vi "Sub Super Duper_2014 05 30_JWb.vi"(0 "VISA resource name":refnum<visa-resource-name>="GPIB0::17::INSTR", 1 "Sample Properties:":T9 {"Date Created" format="%<%Y/%m/%d>T"}, 2 "Gated SMU4 is...":bool, 3 "TRF Cluster":T10={"Step 4"=-38.0, "# of Loops"=1.0, "Transfer 2"=FALSE, "Start 4"=-2.0, "Total Points 2"=2, "Start 3"=40.0, "Stop 2"=-40.0, "Step 3"=-1.0, "Loop Step"=0.0, "Integration Time 3"=0, "Loop Wait"=0.0, "First Step"=0.0} {"Loop Wait" format="%<%H:%M:%S>t"; "Integration Time 3" scale=0.0..2.0; "Step 3" format="%.2f"; "Stop 2" format="%.2f"; "Start 3" format="%.2f"; "Start 4" format="%.2f"; "Step 4" format="%.2f"}, 4 "TSP Cluster":T11={"Transport"=FALSE, "Start 2"=0.0, "Stop 3"=-60.0, "Step 2"=-1.0, "Start"=0.0, "Step"=-10.0, "Total Points"=7, "Integration Time"=0} {"Integration Time" scale=0.0..2.0; "Step" format="%.2f"; "Start" format="%.2f"; "Step 2" format="%.2f"; "Stop 3" format="%.2f"; "Start 2" format="%.2f"}, 5 "Compliance Cluster":T6={"Var1 sweep settings"={"sweep spacing (linear: 0)"=0, "sweep mode"=FALSE, "compliance (V)"=100.0, "compliance (A)"=0.001}, "Var1 sweep settings 2"={"sweep spacing (linear: 0)"=0, "sweep mode"=FALSE, "compliance (V)"=100.0, "compliance (A)"=0.001}, "Var2 step settings 2"={"compliance (A)"=0.001, "compliance (V)"=100.0}, "Var2 step settings"={"compliance (A)"=0.001, "compliance (V)"=100.0}} {"Var2 step settings"."compliance (V)" format="%.2f"; "Var2 step settings"."compliance (A)" format="%^.2e"; "Var2 step settings 2"."compliance (V)" format="%.2f"; "Var2 step settings 2"."compliance (A)" format="%^.2e"; "Var1 sweep settings 2"."compliance (A)" format="%^.2e"; "Var1 sweep settings 2"."compliance (V)" format="%.2f"; "Var1 sweep settings 2"."sweep spacing (linear: 0)" items=["linear", "log 10", "log 25", "log 50"]; "Var1 sweep settings"."compliance (A)" format="%^.2e"; "Var1 sweep settings"."compliance (V)" format="%.2f"; "Var1 sweep settings"."sweep spacing (linear: 0)" items=["linear", "log 10", "log 25", "log 50"]}, 6 "Light Bathe Cluster":T2={"TG to BG:  "=FALSE, "TG to BG Durration"=120.0, "TRF to TSP:   "=FALSE, "TRF to TSP Duration"=120.0, "Post Measure: "=FALSE, "TG to BG (TSP):"=FALSE, "TG to BG Durration 3"=120.0} {"TG to BG Durration 3" format="%<%H:%M:%S>t"; "TRF to TSP Duration" format="%<%H:%M:%S>t"; "TG to BG Durration" format="%<%H:%M:%S>t"}, 7 "error in":errorcluster, 8 "Saved Folder:":path=path "C:/1DATA/2011", 9 "Wait Cluster":T5 {"Wait Time (s)" format="%.1g"; "Wait Countdown" format="%<%H:%M:%S%1u>t"}, 11 "TG Dielectric Prop":T1, 13 "Stop \nCountdown":bool, 15 "Loop Count":dbl, 16 "Gate Current Cluster":T3={"Gate Current (TSP)"={"Y2 axis on/off"=FALSE, "MINIMUM"=0.0, "MAXIMUM"=1.0, "Variable name"="Ig", "LIN or LOG axis"="LIN"}, "Gate Current (TRF)"={"Y2 axis on/off"=FALSE, "MINIMUM"=0.0, "MAXIMUM"=1.0, "Variable name"="Ig", "LIN or LOG axis"="LIN"}} {"Gate Current (TSP)"."MAXIMUM" format="%.9f"; "Gate Current (TSP)"."MINIMUM" format="%.9f"; "Gate Current (TRF)"."MAXIMUM" format="%.9f"; "Gate Current (TRF)"."MINIMUM" format="%.9f"}, 17 "Dielectric Constant (BG)":dbl) -> (12 "Status Indicator":bool, 14 "Vt Cluster":T4 {"Id Max" format="%.3g"; "Vt Max" format="%.3g"; "Vt Min" format="%.3g"; "Vt Ratio" format="%.3g"}, 20 "VISA resource name out":refnum<visa-resource-name>, 21 "TRF Path":path, 23 "TSP Path":path, 24 "Graph Cluster":T7, 25 "Char Cluster":T8 {"Mobility-Lin" format="%#_4e"; "On/Off" format="%#_4e"; "Mobility-Sat" format="%#_4e"}, 27 "error out":errorcluster)   [LabVIEW 2012]
uses:
  <vilib>/Platform/TimedLoop/XDataNode/wakeup.ctl
  <vilib>/Platform/TimedLoop/XDataNode/XDNodeRunTimeDep.lvlib
  <vilib>/Platform/TimedLoop/XDataNode/nitl_modes.ctl
  <vilib>/Platform/TimedLoop/XDataNode/timing_clust.ctl
  <vilib>/Platform/TimedLoop/XDataNode/XDataNode.xnode
panel:
  in  "Ambient Temp (Y/N) 2":bool=TRUE
  in  "Ambient Temp (Y/N)":bool=TRUE
  out "LKG Path":path
  # "Vg Sweep"
  # "Vd Step"
  # "Loops and Integration Time"
  # "Device Characteristics"
  # "Light Bath is..."
  # "Duration (hh:mm:ss)"
  # "Sample Properties:"
  # "%"
  # "nm"
  # "Device Properties:"
  # "um"
  # "um"
  # "Vg Step"
  # "Vd Step"
  # "Integration Time"
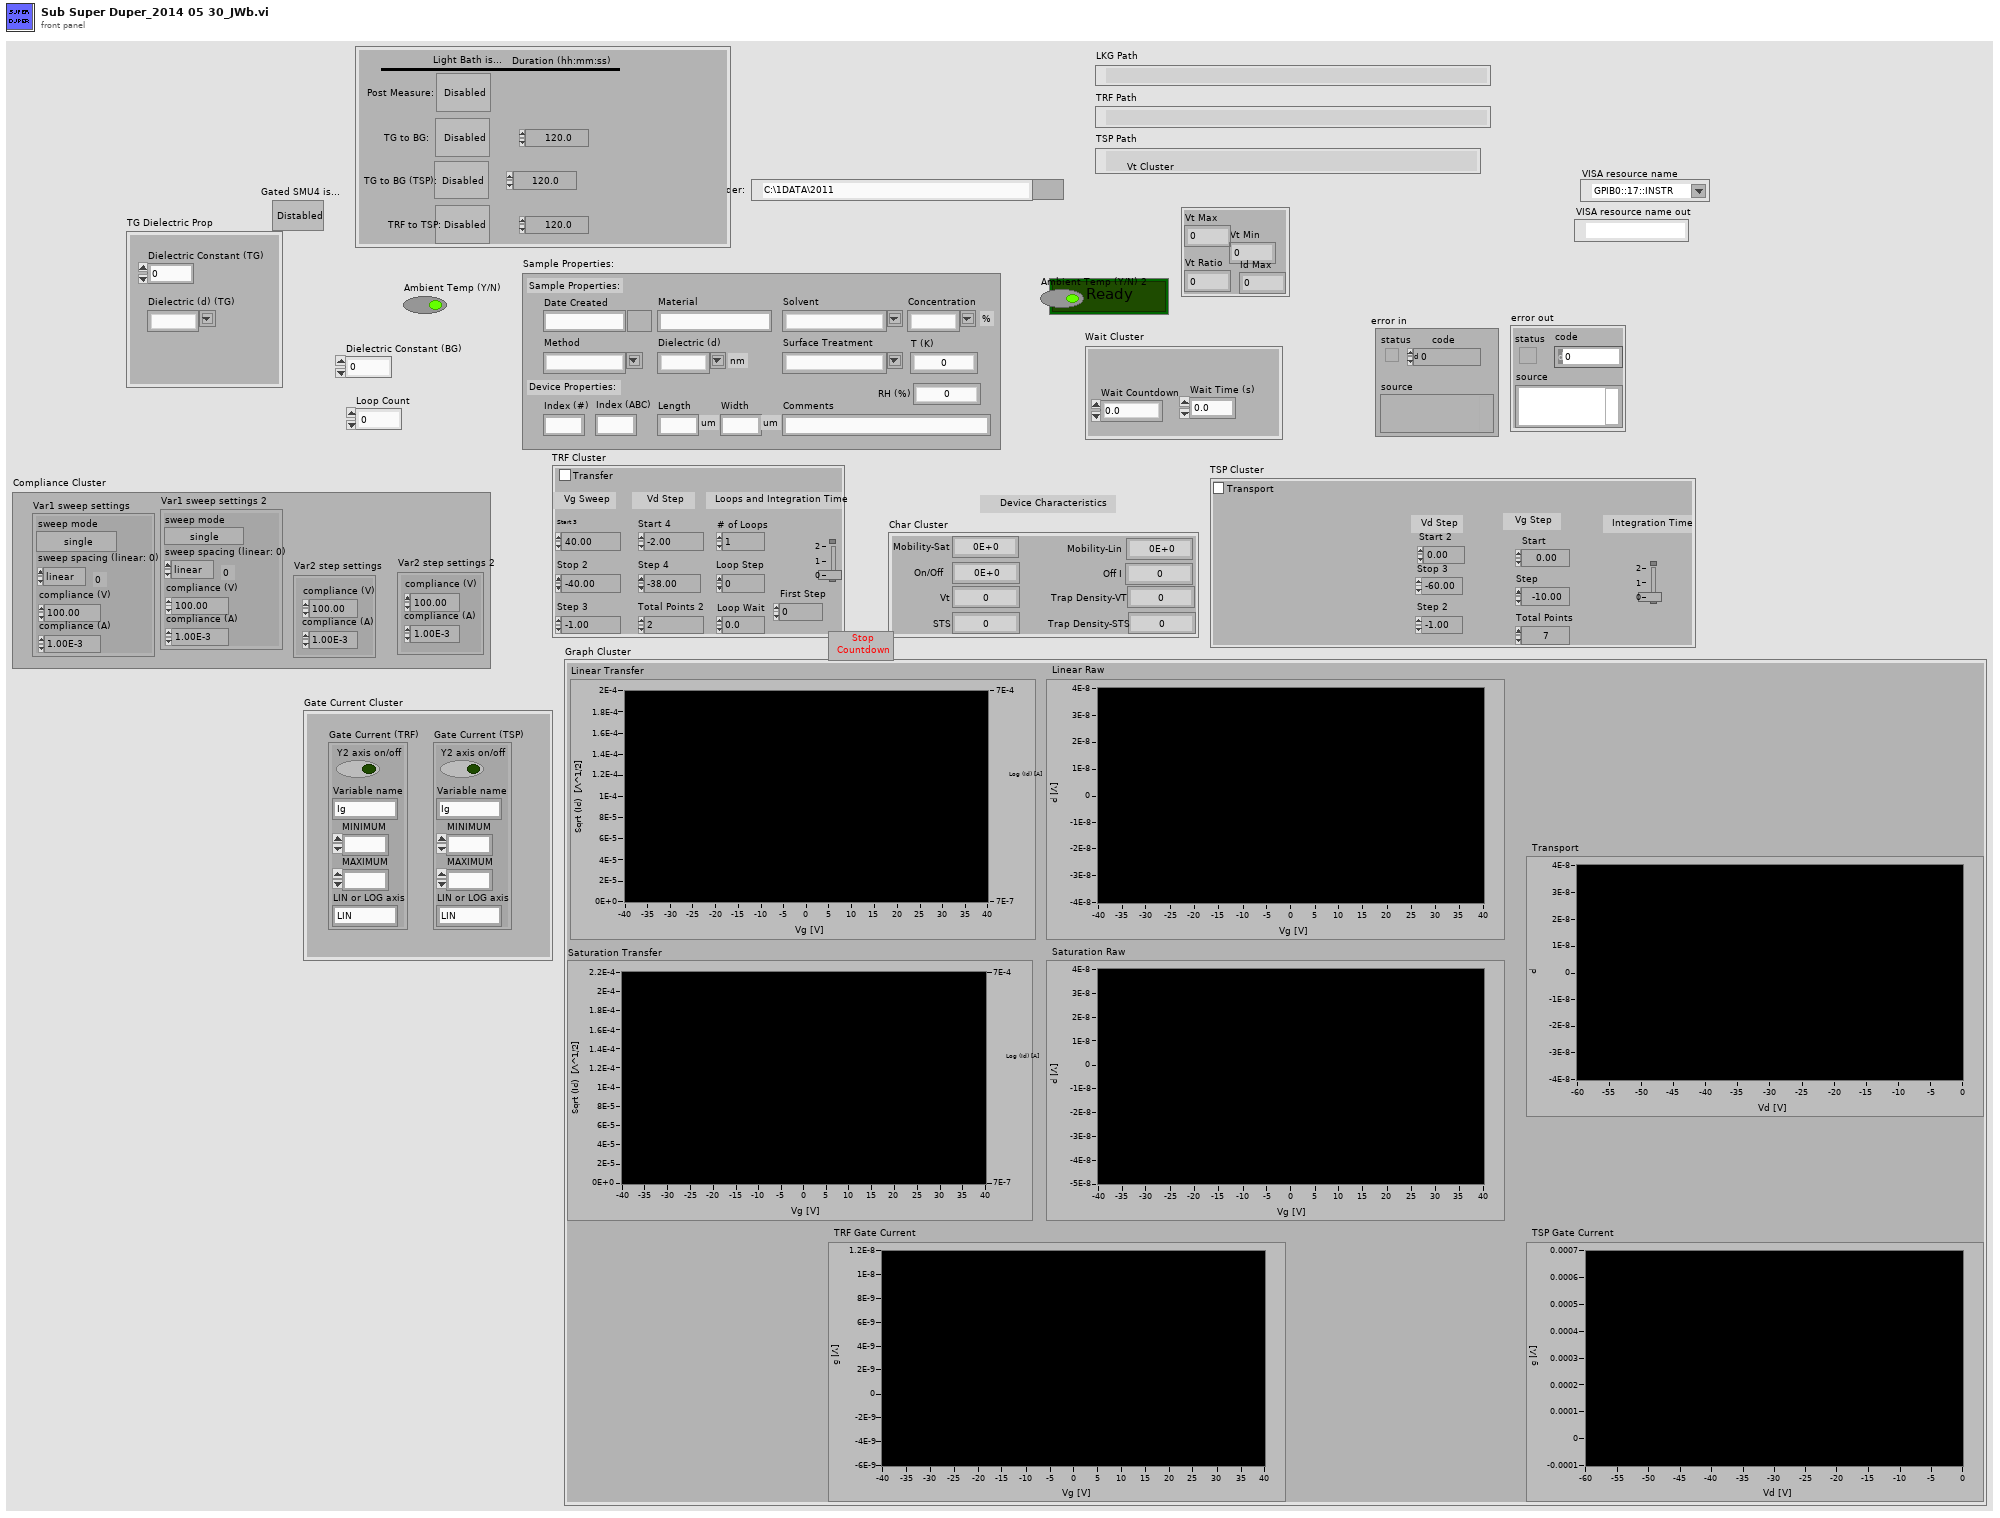
[diagram p1: front panel]
types:
  T1 = cluster{"Dielectric Constant (TG)":dbl, "Dielectric (d) (TG)":string}
  T2 = cluster{"TG to BG:  ":bool, "TG to BG Durration":dbl, "TRF to TSP:   ":bool, "TRF to TSP Duration":dbl, "Post Measure: ":bool, "TG to BG (TSP):":bool, "TG to BG Durration 3":dbl}
  T3 = cluster{"Gate Current (TSP)":cluster{"Y2 axis on/off":bool, "MINIMUM":ext, "MAXIMUM":ext, "Variable name":string, "LIN or LOG axis":string}, "Gate Current (TRF)":cluster{"Y2 axis on/off":bool, "MINIMUM":ext, "MAXIMUM":ext, "Variable name":string, "LIN or LOG axis":string}}
  T4 = cluster{"Vt Max":i32, "Vt Min":i32, "Vt Ratio":i32, "Id Max":i32}
  T5 = cluster{"Wait Countdown":dbl, "Wait Time (s)":dbl}
  T6 = cluster{"Var1 sweep settings":cluster{"sweep spacing (linear: 0)":u16, "sweep mode":bool, "compliance (V)":dbl, "compliance (A)":dbl}, "Var1 sweep settings 2":cluster{"sweep spacing (linear: 0)":u16, "sweep mode":bool, "compliance (V)":dbl, "compliance (A)":dbl}, "Var2 step settings 2":cluster{"compliance (A)":dbl, "compliance (V)":dbl}, "Var2 step settings":cluster{"compliance (A)":dbl, "compliance (V)":dbl}}
  T7 = cluster{"Linear Transfer":cluster{dbl[], "trace":dbl[]}[], "Linear Raw":cluster{dbl[], dbl[]}[], "Saturation Transfer":cluster{dbl[], "trace":dbl[]}[], "Saturation Raw":cluster{dbl[], dbl[]}[], "Transport":cluster{dbl[], dbl[]}[], "TRF Gate Current":cluster{dbl[], dbl[]}[], "TSP Gate Current":cluster{dbl[], dbl[]}[]}
  T8 = cluster{"Mobility-Sat":dbl, "Mobility-Lin":dbl, "On/Off ":dbl, "Off I":dbl, "Vt":dbl, "STS":dbl, "Trap Density-VT":dbl, "Trap Density-STS":dbl}
  T9 = cluster{"Date Created":timestamp, "Material":string, "Solvent":string, "Concentration":string, "Method":string, "Dielectric (d)":string, "Index (#)":string, "Index (ABC)":string, "Length":string, "Width":string, "Surface Treatment":string, "Comments":string, "T (K)":dbl, "RH (%)":dbl}
  T10 = cluster{"Step 4":dbl, "# of Loops":dbl, "Transfer 2":bool, "Start 4":dbl, "Total Points 2":u16, "Start 3":dbl, "Stop 2":dbl, "Step 3":dbl, "Loop Step":dbl, "Integration Time 3":u32, "Loop Wait":dbl, "First Step":dbl}
  T11 = cluster{"Transport":bool, "Start 2":dbl, "Stop 3":dbl, "Step 2":dbl, "Start":dbl, "Step":dbl, "Total Points":u16, "Integration Time":u32}
  T12 = cluster{"Vname":string, "Vname 2":string, "Vname 3":string, "Vname 4":string, "Iname":string, "Iname 2":string, "Iname 3":string, "Iname 4":string, "Mode":u16, "Mode 2":u16, "Mode 3":u16, "Mode 4":u16, "Function":u16, "Function 2":u16, "Function 3":u16, "Function 4":u16, "Value (V or A)":dbl, "Value (Either V or A) 2":dbl, "Value (Either V or A) 3":dbl, "Value (Either V or A) 4":dbl}
  T13 = typedef "XDNodeRunTimeDep.lvlib/timing_clust.ctl" = cluster{"Expected End [f-1]":u64, "Actual End [f-1]":u64, "Finished Late? [f-1]":bool, "Expected End [i-1]":u64, "Actual End [i-1]":u64, "Finished Late? [i-1]":bool, "Expected Start [i]":u64, "Actual Start [i]":u64, "Expected Start [f]":u64, "Actual Start [f]":u64, "Source Name":string, "Structure Name":string, "Period":i64, "Deadline":i64, "Offset":i64, "Start":i64, "Priority":i32, "Timeout":i32, "Mode":T14, "Wakeup Reason":T15, "Error":errorcluster, "Source Type":string, "Secondary Source Type":string, "Global End Time":u64, "Global Start Time":u64, "Frame Duration":u64, "Iteration Duration":u64, "Assigned CPU":i32, "I/O Scan Engine Mode":u32}
  T14 = typedef "XDNodeRunTimeDep.lvlib/nitl_modes.ctl" = enum32{"No Change", "Process missed periods, maintain original phase", "Discard missed periods, maintain original phase", "Process missed periods, ignore original phase", "Discard missed periods, ignore original phase"}
  T15 = typedef "XDNodeRunTimeDep.lvlib/wakeup.ctl" = enum32{"Normal", "Aborted", "Asynchronous wakeup", "Timing source error", "Timed loop error", "Timeout"}
  T16 = cluster{"Vt Max":i32, "Vt Min":i32, "Vt Ratio":i32, "Id Max":dbl}
  T17 = cluster{"Mobility-Sat":dbl, "Mobility-Lin":dbl, "On/Off Current":dbl, "Off I":dbl, "Vt":dbl, "STS":dbl, "Trap Density-VT":dbl, "Trap Density-STS":dbl}
  T18 = cluster{"sweep spacing (linear: 0)":u16, "sweep mode":bool, "compliance (V)":dbl, "compliance (A)":dbl}
  T19 = cluster{"compliance (A)":dbl, "compliance (V)":dbl}
  T20 = cluster{"Y2 axis on/off":bool, "MINIMUM":ext, "MAXIMUM":ext, "Variable name":string, "LIN or LOG axis":string}
  T21 = cluster{"Start 2":dbl, "Stop 3":dbl, "Step 2":dbl, "sweep spacing (linear: 0)":u16, "sweep mode":bool, "compliance (V)":dbl, "compliance (A)":dbl}
  T22 = cluster{"compliance (A)":dbl, "compliance (V)":dbl, "Start":dbl, "Total Points":u16, "Step":dbl}
  T23 = cluster{"Transport":cluster{dbl[], dbl[]}[], "Gate Current":cluster{dbl[], dbl[]}[]}
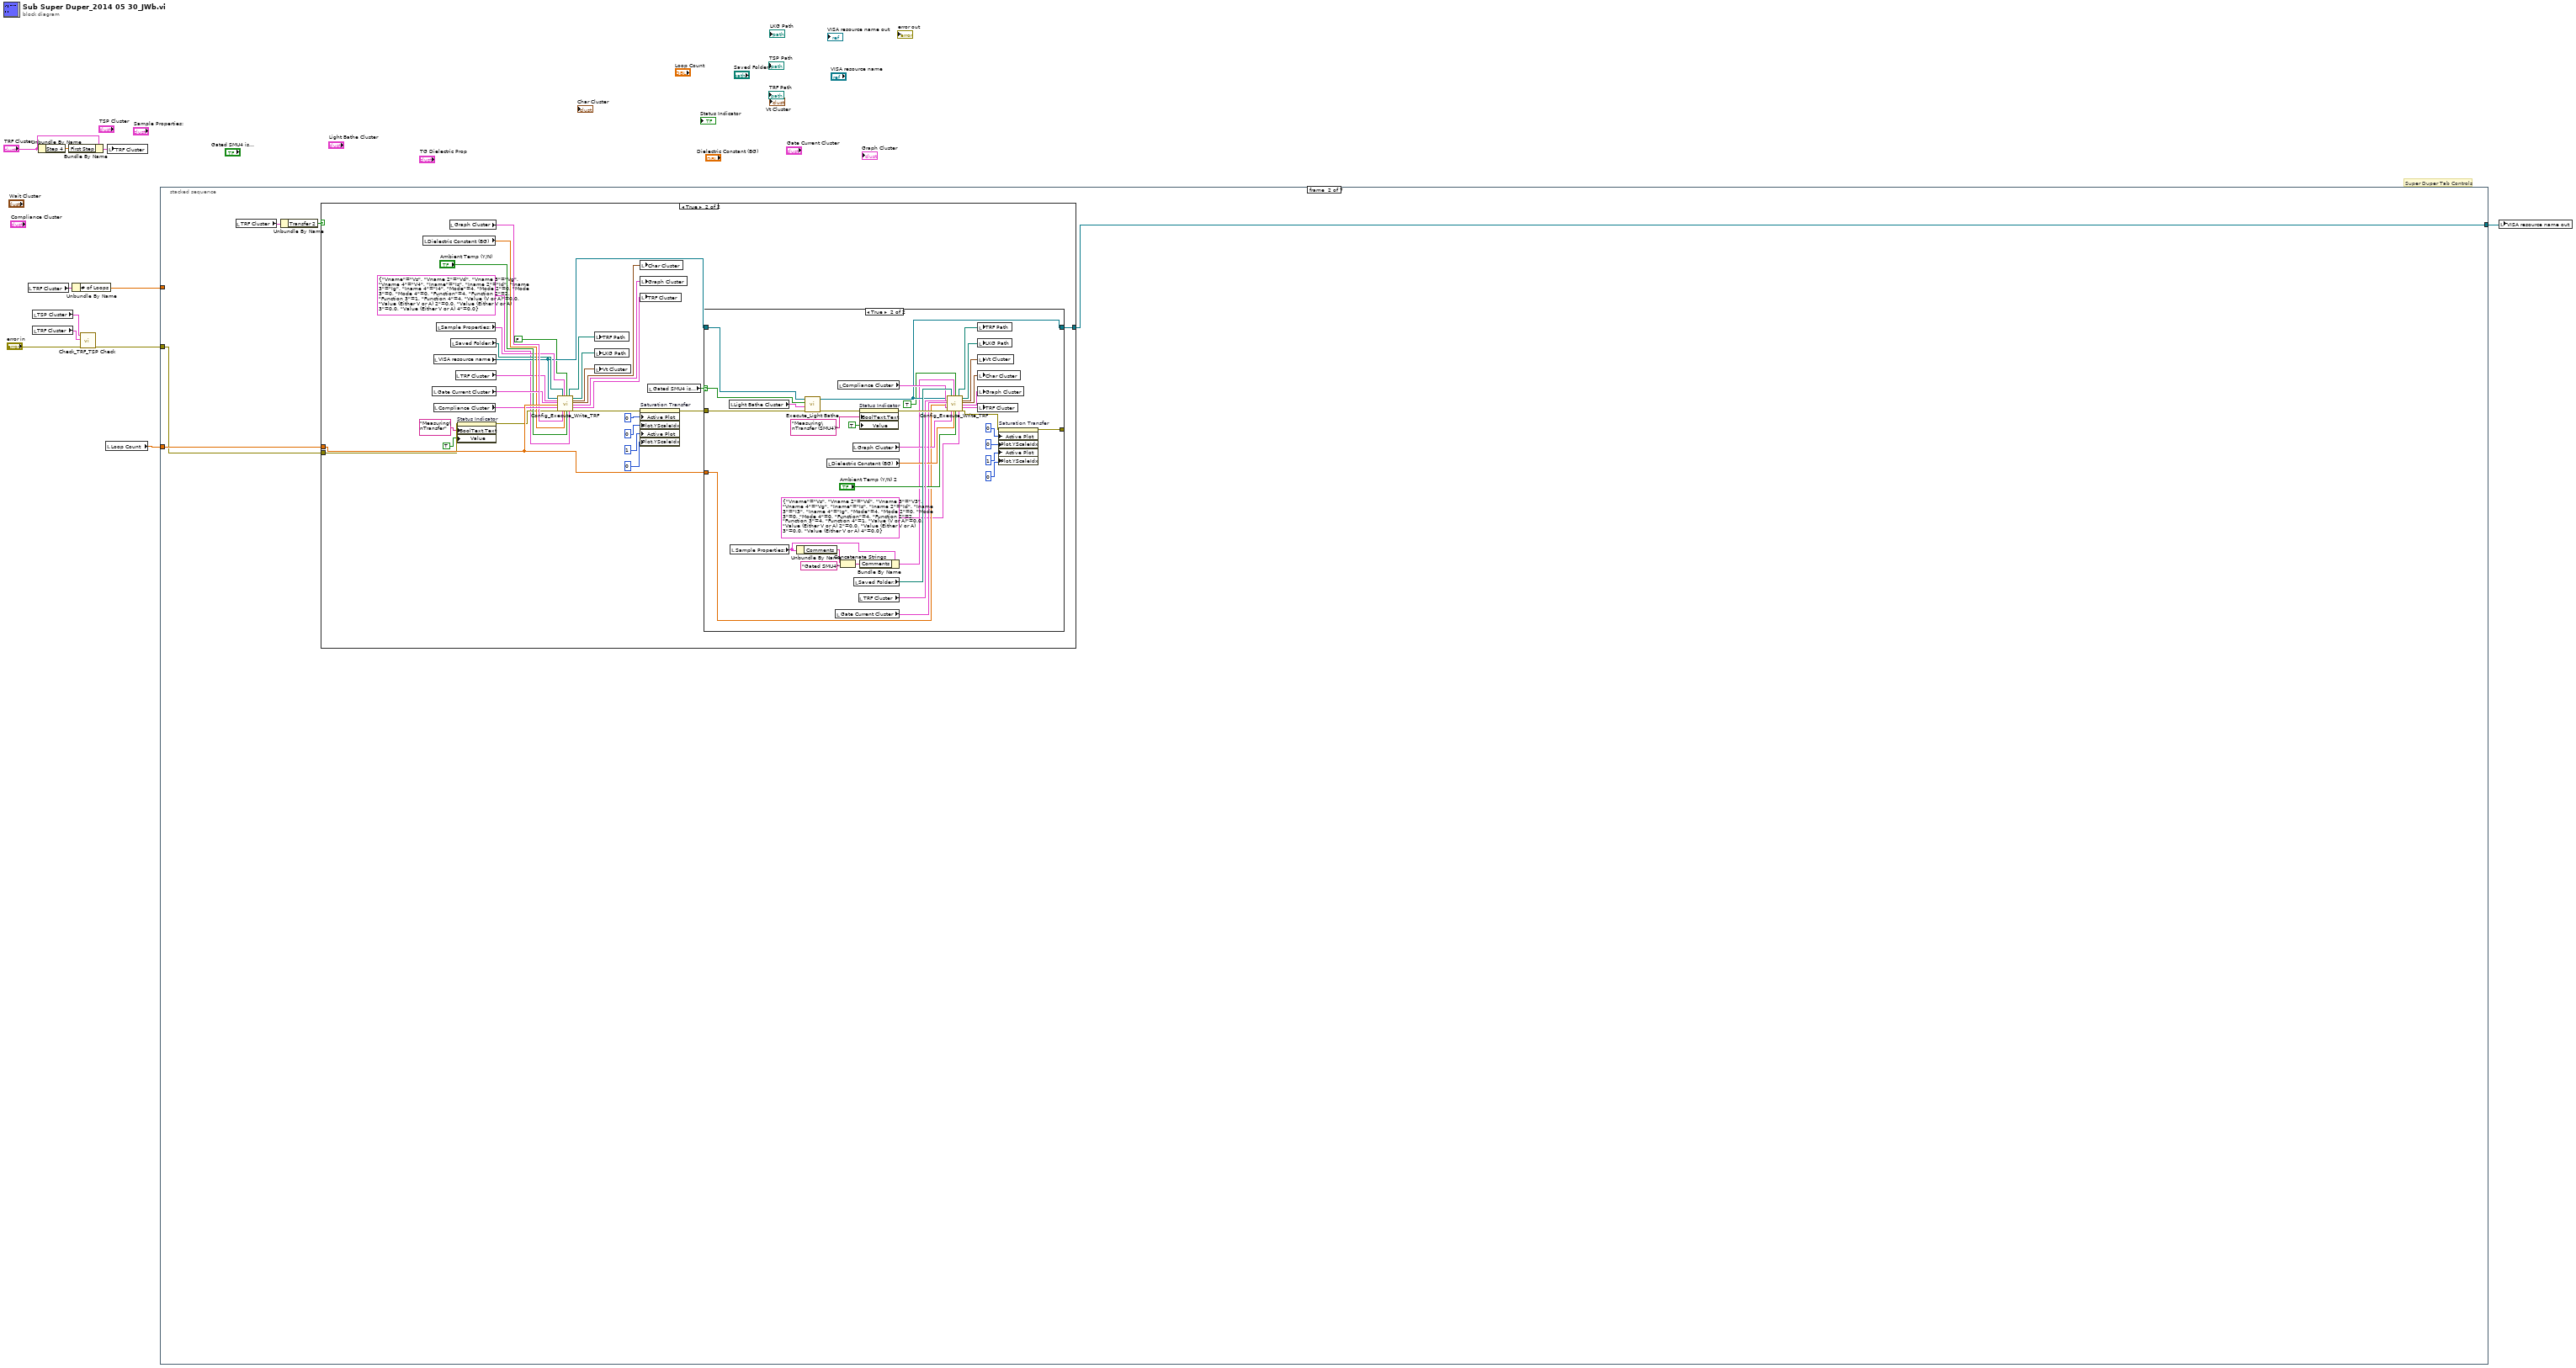
[diagram p0: block diagram]
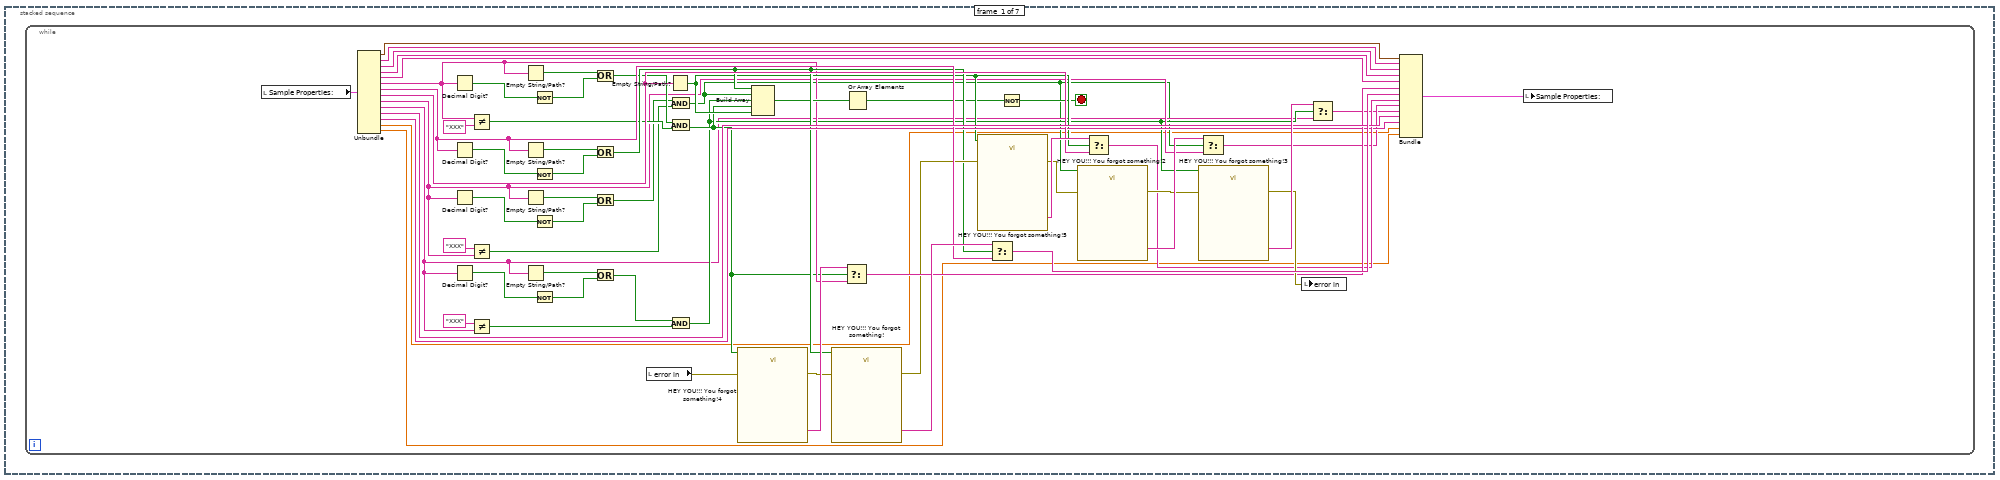
[diagram p2: hidden frame]
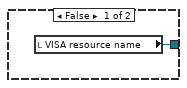
[diagram p3: hidden frame]
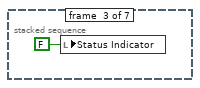
[diagram p5: hidden frame]
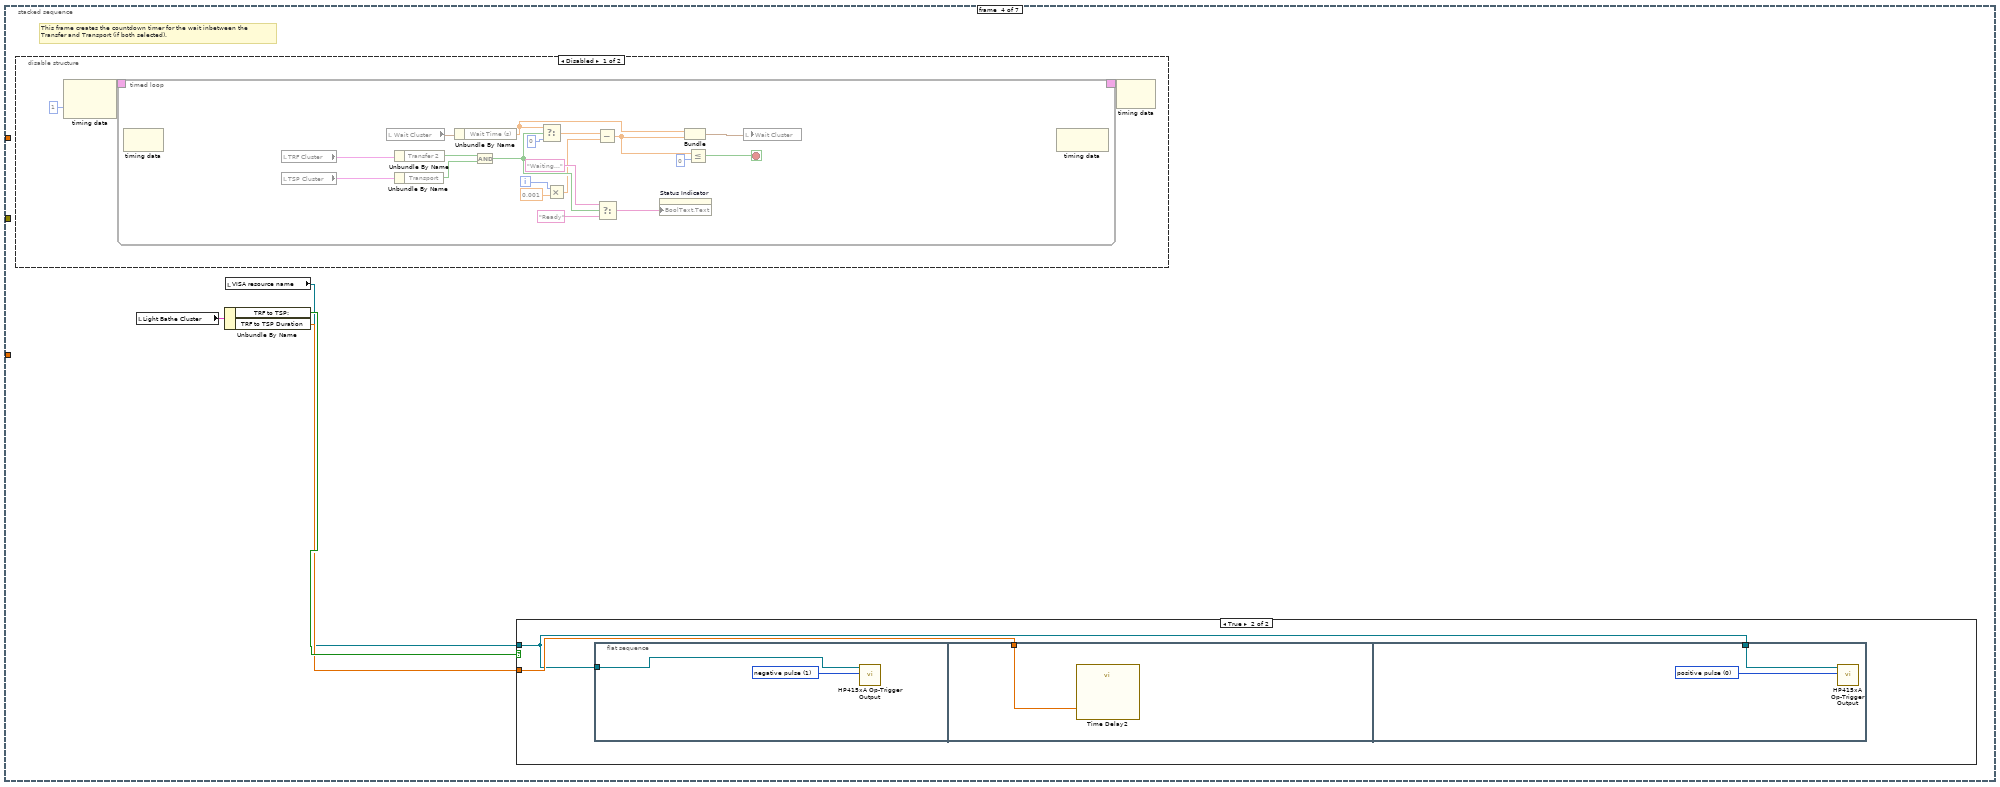
[diagram p6: hidden frame]
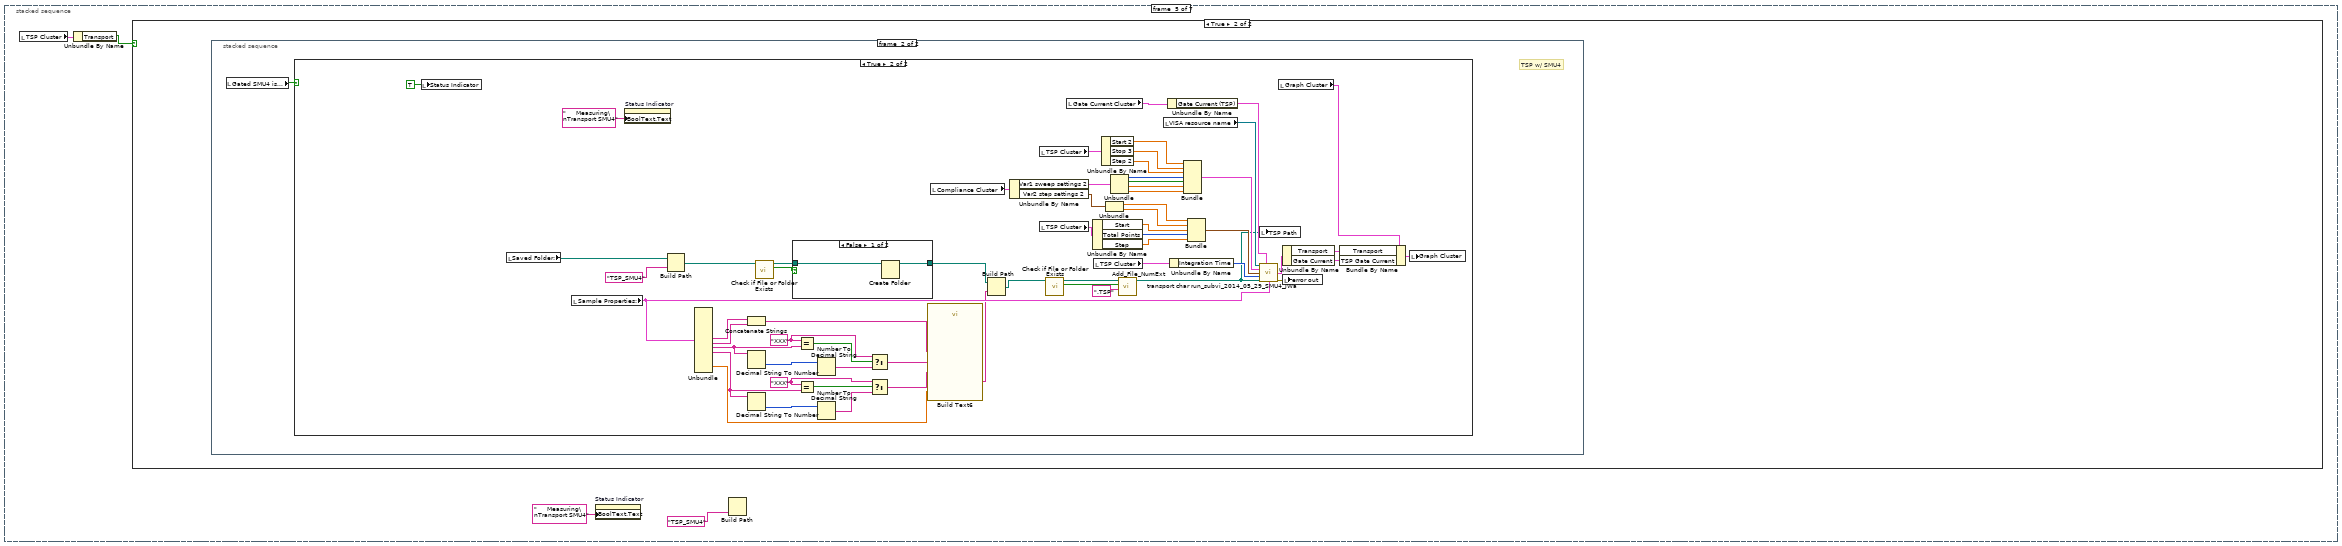
[diagram p9: hidden frame]
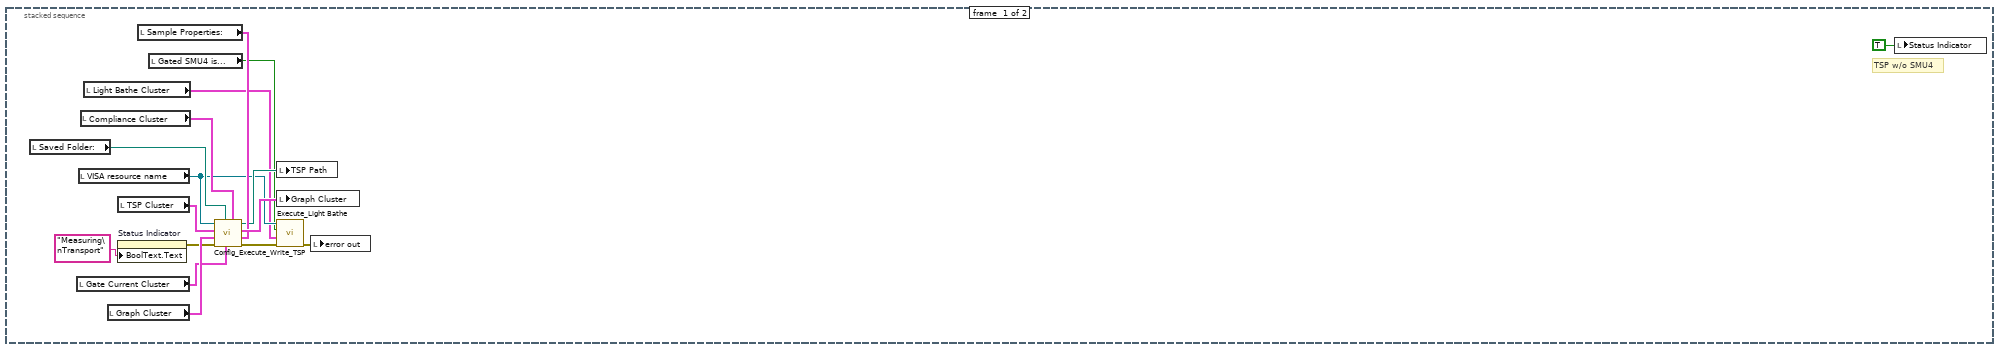
[diagram p11: hidden frame]
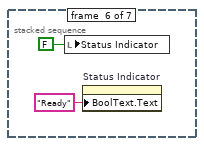
[diagram p14: hidden frame]
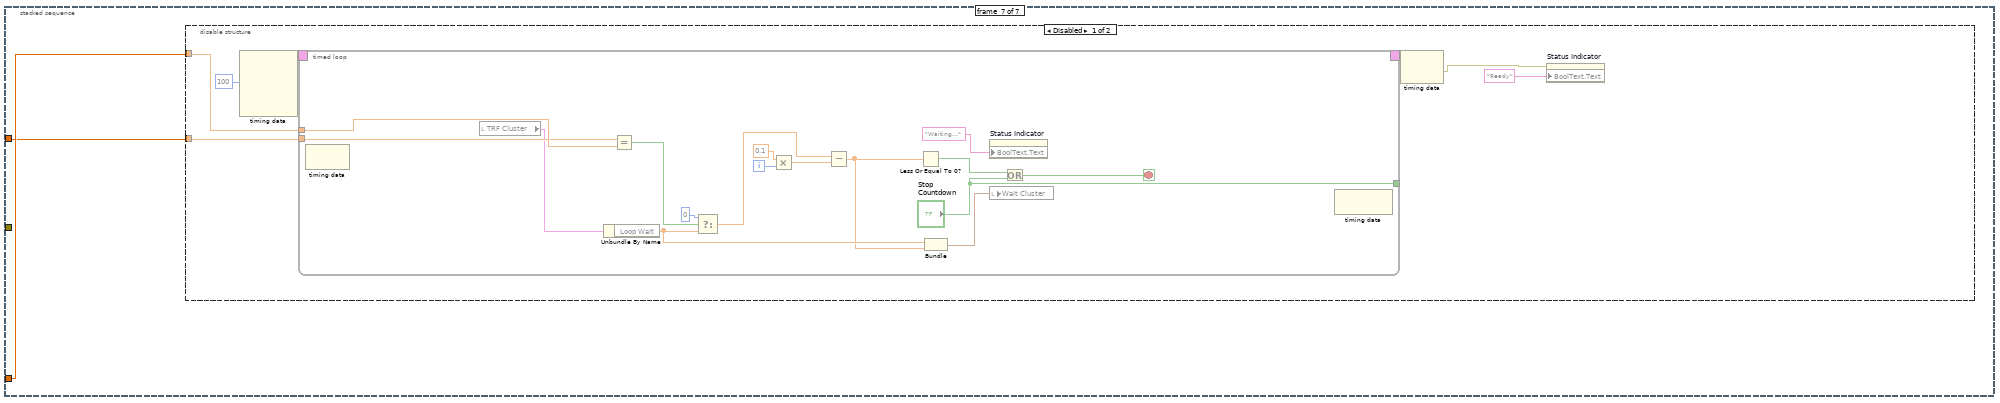
[diagram p15: hidden frame]
diagram:
  # "Super Duper Tab Controls"
  n1 = local read "TRF Cluster"() -> (w8:T10)
  n2 = local read "TSP Cluster"() -> (w4:T11)
  n3 = local read "TRF Cluster"() -> (w3:T10)
  n4 = Unbundle By Name("TRF Cluster") -> ("Step 4"=w9:dbl)
  n5 = Bundle By Name(cluster="TRF Cluster", "First Step"=w9) -> (w11:T10)
  n6 = Unbundle By Name(w8) -> ("# of Loops"=w7:dbl)
  n7 = call "Check_TRF_TSP Check.vi"("error in"="error in", "TRF Cluster"=w3, "TSP Cluster"=w4) -> ("error out"=w1:errorcluster)  [unwired: 8 in]
  n8 = local read "Loop Count"() -> (w5:dbl)
  n9 = local write "TRF Cluster"(w11) -> ()
  n10 = stacked-sequence {
    tunnel: w5 -> [_ w77 _ _ _ _ w276]
    tunnel: w7 -> [_ _ _ _ _ _ w275]
    tunnel: [_ w74 _ _ _ _ _] -> w6
    tunnel: w1 -> [_ w73 _ _ _ _ _]
    frame #0 {
      n11 = while {
        stop <- w38 stop-if-true
        n12 = local read "Sample Properties:"() -> (w67:T9)
        n13 = Unbundle(w67) -> ("Date Created"=w68:timestamp, "Material"=w69:string, "Solvent"=w70:string, "Concentration"=w71:string, "Method"=w72:string, "Dielectric (d)"=w27:string, "Index (#)"=w57:string, "Index (ABC)"=w54:string, "Length"=w22:string, "Width"=w15:string, "Surface Treatment"=w60:string, "Comments"=w52:string, "T (K)"=w13:dbl, "RH (%)"=w12:dbl)
        n14 = Decimal Digit?(1:w27) -> (0:w35:bool)
        n15 = Decimal Digit?(1:w57) -> (0:w48:bool)
        n16 = Decimal Digit?(1:w22) -> (0:w37:bool)
        n17 = Decimal Digit?(1:w15) -> (0:w36:bool)
        n18 = Not Equal?(x=w27, y="XXX") -> (x != y?=w26:bool)
        n19 = Not Equal?(x="XXX", y=w22) -> (x != y?=w21:bool)
        n20 = Not Equal?(x="XXX", y=w15) -> (x != y?=w19:bool)
        n21 = Empty String/Path?(string/path=w27) -> (empty?=w29:bool)
        n22 = Empty String/Path?(string/path=w57) -> (empty?=w56:bool)
        n23 = Empty String/Path?(string/path=w22) -> (empty?=w31:bool)
        n24 = Empty String/Path?(string/path=w15) -> (empty?=w30:bool)
        n25 = Not(x=w35) -> (.not. x?=w32:bool)
        n26 = Not(x=w48) -> (.not. x?=w47:bool)
        n27 = Not(x=w37) -> (.not. x?=w34:bool)
        n28 = Not(x=w36) -> (.not. x?=w33:bool)
        n29 = Or(x=w29, y=w32) -> (x .or. y?=w25:bool)
        n30 = Or(x=w56, y=w47) -> (x .or. y?=w42:bool)
        n31 = Or(x=w31, y=w34) -> (x .or. y?=w20:bool)
        n32 = Or(x=w30, y=w33) -> (x .or. y?=w18:bool)
        n33 = local read "error in"() -> (w44:errorcluster)
        n34 = Empty String/Path?(string/path=w54) -> (empty?=w41:bool)
        n35 = And(x=w20, y=w21) -> (x .and. y?=w14:bool)
        n36 = And(x=w25, y=w26) -> (x .and. y?=w24:bool)
        n37 = And(x=w18, y=w19) -> (x .and. y?=w17:bool)
        n38 = call "HEY YOU!!! You forgot something!4"("Enable"=w24, "error in (no error)"=w44) -> ("Dielectric (d)"=w59:string, "error out"=w43:errorcluster)  [unwired: 15 in, 1 out]
        n39 = Build Array(w42, w14, w17, w24, w41) -> (w40:bool[])
        n40 = call "HEY YOU!!! You forgot something!"("Enable"=w42, "error in (no error)"=w43) -> ("Index (#)"=w66:string, "error out"=w46:errorcluster)  [unwired: 15 in, 1 out]
        n41 = Select(t=w59, s=w24, f=w27) -> (s? t:f=w58:string)
        n42 = Or Array Elements(Boolean array=w40) -> (logical OR=w39:bool)
        n43 = call "HEY YOU!!! You forgot something!5"("Enable"=w41, "error in (no error)"=w46) -> ("Index (ABC)"=w55:string, "error out"=w45:errorcluster)  [unwired: 15 in, 1 out]
        n44 = Select(t=w66, s=w42, f=w57) -> (s? t:f=w63:string)
        n45 = Not(x=w39) -> (.not. x?=w38:bool)
        n46 = call "HEY YOU!!! You forgot something!2"("Enable"=w14, "error in (no error)"=w45) -> ("Length"=w65:string, "error out"=w62:errorcluster)  [unwired: 15 in, 1 out]
        n47 = Select(t=w55, s=w41, f=w54) -> (s? t:f=w53:string)
        n48 = call "HEY YOU!!! You forgot something!3"("Enable"=w17, "error in (no error)"=w62) -> ("Width"=w64:string, "error out"=w61:errorcluster)  [unwired: 15 in, 1 out]
        n49 = Select(t=w65, s=w14, f=w22) -> (s? t:f=w51:string)
        n50 = local write "error in"(w61) -> ()
        n51 = Select(t=w64, s=w17, f=w15) -> (s? t:f=w50:string)
        n52 = Bundle("Date Created"=w68, "Material"=w69, "Solvent"=w70, "Concentration"=w71, "Method"=w72, "Dielectric (d)"=w58, "Index (#)"=w63, "Index (ABC)"=w53, "Length"=w51, "Width"=w50, "Surface Treatment"=w60, "Comments"=w52, "T (K)"=w13, "RH (%)"=w12) -> (w49:T9)  [unwired: 1 in]
        n53 = local write "Sample Properties:"(w49) -> ()
      }
    }
    frame #1 {
      n54 = local read "TRF Cluster"() -> (w75:T10)
      n55 = Unbundle By Name(w75) -> ("Transfer 2"=w76:bool)
      n56 = case shown="True" w76 {
        tunnel: w77 -> [_ w108]
        tunnel: [w78 w107] -> w74
        tunnel: w73 -> [_ w106]
        frame False {
          n57 = local read "VISA resource name"() -> (w78:refnum<visa-resource-name>)
        }
        frame True {
          n58 = local read "Dielectric Constant (BG)"() -> (w93:dbl)
          n59 = local read "Gate Current Cluster"() -> (w94:T3)
          n60 = local read "VISA resource name"() -> (w82:refnum<visa-resource-name>)
          n61 = local read "Compliance Cluster"() -> (w100:T6)
          n62 = local read "Sample Properties:"() -> (w90:T9)
          n63 = local read "Graph Cluster"() -> (w96:T7)
          n64 = local read "Saved Folder:"() -> (w91:path)
          n65 = local read "TRF Cluster"() -> (w86:T10)
          n66 = property on="Status Indicator" class="Bool (strict)"(error in=w106, "BoolText.Text"="Measuring\nTransfer", "Value"=TRUE) -> (error out=w84:errorcluster)  [unwired: 1 in, 1 out]
          n67 = call "Config_Execute_Write_TRF.vi"("VISA Refnum in"=w82, "TRF Cluster in"=w86, "Gate Current Cluster"=w94, "Loop Count"=w108, "Compliance Cluster"=w100, "Error In"=w84, "Saved Folder:"=w91, "Graph Cluster"=w96, "Sample Properties:"=w90, "Dielectric Constant (BG)"=w93, "SMU4? (Y/N)"=FALSE, "Ambient Temp (Y/N)"="Ambient Temp (Y/N)", "SMU Config"=T12 {"Vname"="Vs", "Vname 2"="Vd", "Vname 3"="Vg", "Vname 4"="V4", "Iname"="Is", "Iname 2"="Id", "Iname 3"="Ig", "Iname 4"="I4", "Mode"=4, "Mode 2"=0, "Mode 3"=0, "Mode 4"=0, "Function"=4, "Function 2"=2, "Function 3"=1, "Function 4"=4, "Value (V or A)"=0.0, "Value (Either V or A) 2"=0.0, "Value (Either V or A) 3"=0.0, "Value (Either V or A) 4"=0.0}) -> ("Filepath Out 2"=w89:path, "Filepath Out"=w88:path, "Check Cluster"=w97:T16, "Output"=w98:T17, "Graph Cluster out"=w95:T7, "TRF Cluster out"=w99:T10, "error out"=w87:errorcluster)
          n68 = local write "TRF Path"(w89) -> ()
          n69 = local write "LKG Path"(w88) -> ()
          n70 = local write "Vt Cluster"(w97) -> ()
          n71 = local write "Char Cluster"(w98) -> ()
          n72 = local write "Graph Cluster"(w95) -> ()
          n73 = local write "TRF Cluster"(w99) -> ()
          n74 = property on="Saturation Transfer" class="XYGraph (strict)"(error in=w87, "Active Plot"=0, "Plot.YScaleIdx"=0, "Active Plot"=1, "Plot.YScaleIdx"=0) -> (error out=w83:errorcluster)  [unwired: 1 in, 1 out]
          n75 = local read "Gated SMU4 is..."() -> (w79:bool)
          n76 = case shown="True" w79 {
            selector: w79 -> [_ w111]
            tunnel: w83 -> [w109 w146]
            tunnel: w82 -> [w110 w144]
            tunnel: w108 -> [_ w118]
            tunnel: [w110 w117] -> w107
            tunnel: [w109 w112] -> _
            frame False {
            }
            frame True {
              n77 = local read "Light Bathe Cluster"() -> (w145:T2)
              n78 = local read "Sample Properties:"() -> (w116:T9)
              n79 = Unbundle By Name(w116) -> ("Comments"=w143:string)
              n80 = call "Execute_Light Bathe.vi"("error in (no error)"=w146, "Light Bathe Cluster"=w145, "Gated SMU4 is..."=w111, "VISA Refnum in"=w144) -> ("Error Out"=w119:errorcluster, "VISA Out"=w117:refnum<visa-resource-name>)  [unwired: 6 in]
              n81 = local read "Dielectric Constant (BG)"() -> (w132:dbl)
              n82 = local read "Gate Current Cluster"() -> (w131:T3)
              n83 = local read "Compliance Cluster"() -> (w125:T6)
              n84 = Concatenate Strings(w143, "Gated SMU4" ("string")) -> (w141:string)
              n85 = local read "Graph Cluster"() -> (w129:T7)
              n86 = local read "Saved Folder:"() -> (w134:path)
              n87 = local read "TRF Cluster"() -> (w138:T10)
              n88 = Bundle By Name(cluster=w116, "Comments"=w141) -> (w115:T9)
              n89 = property on="Status Indicator" class="Bool (strict)"(error in=w119, "BoolText.Text"="Measuring\nTransfer (SMU4)", "Value"=TRUE) -> (error out=w140:errorcluster)  [unwired: 1 in, 1 out]
              n90 = call "Config_Execute_Write_TRF.vi"("VISA Refnum in"=w117, "TRF Cluster in"=w138, "Gate Current Cluster"=w131, "Loop Count"=w118, "Compliance Cluster"=w125, "Error In"=w140, "Saved Folder:"=w134, "Graph Cluster"=w129, "Sample Properties:"=w115, "Dielectric Constant (BG)"=w132, "SMU4? (Y/N)"=TRUE, "Ambient Temp (Y/N)"="Ambient Temp (Y/N) 2", "SMU Config"=T12 {"Vname"="Vs", "Vname 2"="Vd", "Vname 3"="V3", "Vname 4"="Vg", "Iname"="Is", "Iname 2"="Id", "Iname 3"="I3", "Iname 4"="Ig", "Mode"=4, "Mode 2"=0, "Mode 3"=0, "Mode 4"=0, "Function"=4, "Function 2"=2, "Function 3"=4, "Function 4"=1, "Value (V or A)"=0.0, "Value (Either V or A) 2"=0.0, "Value (Either V or A) 3"=0.0, "Value (Either V or A) 4"=0.0}) -> ("Filepath Out 2"=w135:path, "Filepath Out"=w136:path, "Check Cluster"=w128:T16, "Output"=w127:T17, "Graph Cluster out"=w130:T7, "TRF Cluster out"=w126:T10, "error out"=w137:errorcluster)
              n91 = local write "TRF Path"(w135) -> ()
              n92 = local write "LKG Path"(w136) -> ()
              n93 = local write "Vt Cluster"(w128) -> ()
              n94 = local write "Char Cluster"(w127) -> ()
              n95 = local write "Graph Cluster"(w130) -> ()
              n96 = local write "TRF Cluster"(w126) -> ()
              n97 = property on="Saturation Transfer" class="XYGraph (strict)"(error in=w137, "Active Plot"=0, "Plot.YScaleIdx"=0, "Active Plot"=1, "Plot.YScaleIdx"=0) -> (error out=w112:errorcluster)  [unwired: 1 in, 1 out]
            }
          }
        }
      }
    }
    frame #2 {
      n98 = local write "Status Indicator"(FALSE) -> ()
    }
    frame #3 {
      # "This frame creates the countdown timer for the wait inbetween the\nTransfer and Transport (if both selected)."
      n99 = disable-structure shown="Disabled" {
        frame Disabled {
          n100 = node-c288(1) -> (w161:T13)  [unwired: 1 in]
          n101 = timed-loop {
            timing: w161 -> [_]
            timing-out: [_] -> w160
            i -> [w172]
            stop <- w173 stop-if-true
            n102 = node-c288() -> ()  [unwired: 1 in, 1 out]
            n103 = local read "TRF Cluster"() -> (w166:T10)
            n104 = local read "TSP Cluster"() -> (w167:T11)
            n105 = local read "Wait Cluster"() -> (w165:T5)
            n106 = Unbundle By Name(w166) -> ("Transfer 2"=w169:bool)
            n107 = Unbundle By Name(w167) -> ("Transport"=w168:bool)
            n108 = Unbundle By Name(w165) -> ("Wait Time (s)"=w163:dbl)
            n109 = And(x=w169, y=w168) -> (x .and. y?=w177:bool)
            n110 = Select(t=w163, s=w177, f=0) -> (s? t:f=w175:dbl)
            n111 = Multiply(x=w172, y=0.001) -> (x*y=w170:dbl)
            n112 = Subtract(x=w175, y=w170) -> (x-y=w164:dbl)
            n113 = Select(t="Waiting...", s=w177, f="Ready") -> (s? t:f=w179:string)
            n114 = property on="Status Indicator" class="Bool (strict)"("BoolText.Text"=w179) -> ()  [unwired: 2 in, 2 out]
            n115 = Bundle("Wait Time (s)"=w163, w164) -> (w162:cluster{"Wait Time (s)":dbl, dbl})  [unwired: 1 in]
            n116 = Less Or Equal?(x=w164, y=0) -> (x <= y?=w173:bool)
            n117 = local write "Wait Cluster"(w162) -> ()
            n118 = node-c288() -> ()  [unwired: 1 in, 1 out]
          }
          n119 = node-c288(w160) -> ()  [unwired: 1 out]
        }
        frame Enabled {
        }
      }
      n120 = local read "Light Bathe Cluster"() -> (w148:T2)
      n121 = Unbundle By Name(w148) -> ("TRF to TSP:"=w151:bool, "TRF to TSP Duration"=w150:dbl)
      n122 = local read "VISA resource name"() -> (w149:refnum<visa-resource-name>)
      n123 = case shown="True" w151 {
        tunnel: w150 -> [_ w153]
        tunnel: w149 -> [_ w152]
        frame False {
        }
        frame True {
          n124 = flat-sequence {
            tunnel: w152 -> [w154]
            tunnel: w153 -> [w156]
            tunnel: w152 -> [w157]
            frame #0 {
              w155 = u32 1 items=["positive pulse  ", "negative pulse  ", "level high  ", "level low  "] ("trigger signal")
              n125 = call "HP415xA Op-Trigger Output.vi"("trigger signal"=w155, "VISA session"=w154) -> ()  [unwired: 2 in, 1 out]
            }
            frame #1 {
              n126 = call "Time Delay2"("Delay Time (s)"=w156) -> ()  [unwired: 10 in, 1 out]
            }
            frame #2 {
              w158 = u32 0 items=["positive pulse  ", "negative pulse  ", "level high  ", "level low  "] ("trigger signal")
              n127 = call "HP415xA Op-Trigger Output.vi"("trigger signal"=w158, "VISA session"=w157) -> ()  [unwired: 2 in, 1 out]
            }
          }
        }
      }
    }
    frame #4 {
      n128 = local read "TSP Cluster"() -> (w191:T11)
      n129 = Unbundle By Name(w191) -> ("Transport"=w190:bool)
      n130 = case shown="True" w190 {
        frame False {
        }
        frame True {
          n131 = stacked-sequence {
            frame #0 {
              # "TSP w/o SMU4"
              n132 = local read "Saved Folder:"() -> (w201:path)
              n133 = local read "Gate Current Cluster"() -> (w202:T3)
              n134 = local read "VISA resource name"() -> (w196:refnum<visa-resource-name>)
              n135 = local read "Compliance Cluster"() -> (w205:T6)
              n136 = local read "Light Bathe Cluster"() -> (w194:T2)
              n137 = local read "Graph Cluster"() -> (w204:T7)
              n138 = local read "TSP Cluster"() -> (w198:T11)
              n139 = property on="Status Indicator" class="Bool (strict)"("BoolText.Text"="Measuring\nTransport") -> (error out=w197:errorcluster)  [unwired: 2 in, 1 out]
              n140 = local read "Sample Properties:"() -> (w200:T9)
              n141 = local read "Gated SMU4 is..."() -> (w195:bool)
              n142 = call "Config_Execute_Write_TSP.vi"("Sample Properties:"=w200, "Compliance Cluster"=w205, "Gate Current Cluster"=w202, "Saved Folder:"=w201, "error In"=w197, "Graph Cluster in"=w204, "TSP Cluster"=w198, "VISA Refnum in"=w196) -> ("error Out"=w193:errorcluster, "Graph Cluster out"=w203:T7, "Filepath Out"=w199:path)
              n143 = local write "TSP Path"(w199) -> ()
              n144 = local write "Graph Cluster"(w203) -> ()
              n145 = call "Execute_Light Bathe.vi"("error in (no error)"=w193, "Light Bathe Cluster"=w194, "Gated SMU4 is..."=w195, "VISA Refnum in"=w196) -> ("Error Out"=w192:errorcluster)  [unwired: 6 in, 1 out]
              n146 = local write "error out"(w192) -> ()
              n147 = local write "Status Indicator"(TRUE) -> ()
            }
            frame #1 {
              # "TSP w/ SMU4"
              n148 = local read "Gated SMU4 is..."() -> (w208:bool)
              n149 = case shown="True" w208 {
                frame False {
                }
                frame True {
                  w244 = "XXX"
                  w248 = "XXX"
                  n150 = local write "Status Indicator"(TRUE) -> ()
                  n151 = local read "Saved Folder:"() -> (w224:path)
                  n152 = local read "Sample Properties:"() -> (w258:T9)
                  n153 = property on="Status Indicator" class="Bool (strict)"("BoolText.Text"="     Measuring\nTransport SMU4") -> ()  [unwired: 2 in, 2 out]
                  n154 = Build Path(base path=w224, name or relative path="TSP_SMU4") -> (appended path=w237:path)
                  n155 = Unbundle(w258) -> ("Index (#)"=w257:string, "Index (ABC)"=w256:string, "Length"=w249:string, "Width"=w245:string, "T (K)"=w220:dbl)  [unwired: 9 out]
                  n156 = Concatenate Strings(w257, w256) -> (w255:string)
                  n157 = Decimal String To Number(string=w249) -> (number=w252:i32)  [unwired: 2 in, 1 out]
                  n158 = Decimal String To Number(string=w245) -> (number=w251:i32)  [unwired: 2 in, 1 out]
                  n159 = call <vilib>:"Check if File or Folder Exists.vi"("path"=w237) -> ("file or folder exists?"=w239:bool, "dup path"=w238:path)  [unwired: 8 in, 1 out]
                  n160 = case shown="False" w239 {
                    tunnel: w238 -> [w271 w272]
                    tunnel: [w270 w272] -> w236
                    frame False {
                      n161 = Create Folder(path (use dialog)=w271) -> (created path=w270:path)  [unwired: 2 in, 2 out]
                    }
                    frame True {
                    }
                  }
                  n162 = Equal?(x=w248, y=w249) -> (x = y?=w250:bool)
                  n163 = Equal?(x=w244, y=w245) -> (x = y?=w253:bool)
                  n164 = Number To Decimal String(number=w252) -> (decimal integer string=w247:string)  [unwired: 1 in]
                  n165 = Number To Decimal String(number=w251) -> (decimal integer string=w243:string)  [unwired: 1 in]
                  n166 = Select(t=w248, s=w250, f=w247) -> (s? t:f=w246:string)
                  n167 = Select(t=w244, s=w253, f=w243) -> (s? t:f=w242:string)
                  n168 = call "Build Text6"("T"=w220, "Index"=w255, "Length"=w246, "Width"=w242) -> ("Result"=w241:string)  [unwired: 10 in, 1 out]
                  n169 = local read "Compliance Cluster"() -> (w223:T6)
                  n170 = Build Path(base path=w236, name or relative path=w241) -> (appended path=w254:path)
                  n171 = Unbundle By Name(w223) -> ("Var1 sweep settings 2"=w222:T18, "Var2 step settings 2"=w221:T19)
                  n172 = local read "TSP Cluster"() -> (w235:T11)
                  n173 = local read "TSP Cluster"() -> (w226:T11)
                  n174 = call <vilib>:"Check if File or Folder Exists.vi"("path"=w254) -> ("file or folder exists?"=w210:bool, "dup path"=w211:path)  [unwired: 8 in, 1 out]
                  n175 = local read "Gate Current Cluster"() -> (w214:T3)
                  n176 = Unbundle By Name(w226) -> ("Start"=w231:dbl, "Total Points"=w230:u16, "Step"=w229:dbl)
                  n177 = local read "TSP Cluster"() -> (w228:T11)
                  n178 = Unbundle By Name(w235) -> ("Start 2"=w234:dbl, "Stop 3"=w233:dbl, "Step 2"=w232:dbl)
                  n179 = Unbundle(w221) -> ("compliance (A)"=w264:dbl, "compliance (V)"=w263:dbl)
                  n180 = Unbundle(w222) -> ("sweep spacing (linear: 0)"=w269:u16, "sweep mode"=w268:bool, "compliance (V)"=w267:dbl, "compliance (A)"=w266:dbl)
                  n181 = call "Add_File_NumExt.vi"("Extension"=".TSP" ("string"), "file or folder exists?"=w210, "Path In"=w211) -> ("Path Out"=w209:path)  [unwired: 8 in]
                  n182 = local read "VISA resource name"() -> (w225:refnum<visa-resource-name>)
                  n183 = Unbundle By Name(w214) -> ("Gate Current (TSP)"=w213:T20)
                  n184 = Unbundle By Name(w228) -> ("Integration Time"=w227:u32)
                  n185 = Bundle("Start 2"=w234, "Stop 3"=w233, "Step 2"=w232, "sweep spacing (linear: 0)"=w269, "sweep mode"=w268, "compliance (V)"=w267, "compliance (A)"=w266) -> (w265:T21)  [unwired: 1 in]
                  n186 = Bundle("compliance (A)"=w264, "compliance (V)"=w263, "Start"=w231, "Total Points"=w230, "Step"=w229) -> (w262:T22)  [unwired: 1 in]
                  n187 = local write "TSP Path"(w209) -> ()
                  n188 = call "transport char run_subvi_2014_05_29_SMU4_JWa.vi"("VISA session"=w225, "Y2 axis settings"=w213, "Var1 sweep settings"=w265, "Var2 step settings"=w262, "integration time"=w227, "Path"=w209, "Sample Properties:"=w258) -> ("Graph Cluster"=w219:T23, "error?"=w261:errorcluster)  [unwired: 6 in, 1 out]
                  n189 = local read "Graph Cluster"() -> (w218:T7)
                  n190 = Unbundle By Name(w219) -> ("Transport"=w216:cluster{dbl[], dbl[]}[], "Gate Current"=w215:cluster{dbl[], dbl[]}[])
                  n191 = local write "error out"(w261) -> ()
                  n192 = Bundle By Name(cluster=w218, "Transport"=w216, "TSP Gate Current"=w215) -> (w217:T7)
                  n193 = local write "Graph Cluster"(w217) -> ()
                }
              }
            }
          }
        }
      }
      n194 = property on="Status Indicator" class="Bool (strict)"("BoolText.Text"="     Measuring\nTransport SMU4") -> ()  [unwired: 2 in, 2 out]
      n195 = Build Path(name or relative path="TSP_SMU4") -> (base path=w189:path)  [unwired: 1 out]
    }
    frame #5 {
      n196 = local write "Status Indicator"(FALSE) -> ()
      n197 = property on="Status Indicator" class="Bool (strict)"("BoolText.Text"="Ready") -> ()  [unwired: 2 in, 2 out]
    }
    frame #6 {
      n198 = disable-structure shown="Disabled" {
        disable-tunnel: w276 -> [w278 _]
        disable-tunnel: w275 -> [w277 _]
        frame Disabled {
          n199 = node-c288(100) -> (w283:T13)  [unwired: 3 in]
          n200 = timed-loop {
            timing: w283 -> [_]
            timing-out: [_] -> w282
            tunnel: w278 -> [w294]
            tunnel: w277 -> [w293]
            tunnel: ["Stop \nCountdown"] -> _
            i -> [w299]
            stop <- w289 stop-if-true
            n201 = node-c288() -> ()  [unwired: 1 in, 1 out]
            n202 = local read "TRF Cluster"() -> (w288:T10)
            n203 = Unbundle By Name(w288) -> ("Loop Wait"=w286:dbl)
            n204 = Equal?(x=w293, y=w294) -> (x = y?=w295:bool)
            n205 = Select(t=0, s=w295, f=w286) -> (s? t:f=w291:dbl)
            n206 = Multiply(x=0.1, y=w299) -> (x*y=w297:dbl)
            n207 = Subtract(x=w291, y=w297) -> (x-y=w285:dbl)
            n208 = Less Or Equal To 0?(x=w285) -> (x <= 0?=w290:bool)
            n209 = Bundle("Loop Wait"=w286, w285) -> (w287:cluster{"Loop Wait":dbl, dbl})  [unwired: 1 in]
            n210 = property on="Status Indicator" class="Bool (strict)"("BoolText.Text"="Waiting...") -> ()  [unwired: 2 in, 2 out]
            n211 = local write "Wait Cluster"(w287) -> ()
            n212 = Or(x=w290, y="Stop \nCountdown") -> (x .or. y?=w289:bool)
            n213 = node-c288() -> ()  [unwired: 1 in, 1 out]
          }
          n214 = node-c288(w282) -> (w279:errorcluster)
          n215 = property on="Status Indicator" class="Bool (strict)"(error in=w279, "BoolText.Text"="Ready") -> ()  [unwired: 1 in, 2 out]
        }
        frame Enabled {
        }
      }
    }
  }
  n216 = local write "VISA resource name out"(w6) -> ()
